vi "SVM_Crossvalidation_FromFile.vi"(8 "error in (no error)":errorcluster) -> (0 "error out":errorcluster, 3 "Predicted labels":dbl[](array[numeric]))   [LabVIEW 2014]
uses:
  Controls/Kernel.ctl
  Libsvm Wrapper/Controls/svm_kernel_type.ctl
  Controls/Options Training.ctl
  Controls/Parameters C_SVC.ctl
  SubVIs/SVM Cross-Validate C_SVC.vi
  <userlib>/_OpenG.lib/error/error.llb/Filter Error Codes (Array)__ogtk.vi
  Libsvm Wrapper/svm_cross_validation.vi
panel:
  in  "Param":T1={"C"=1.0, "weight_label"=[], "weight"=[]}
  in  "Nr Fold":i32=5 caption="Nr fold (LOO)"
  in  "Options":T2={"cache_size"=500.0, "eps"=0.001, "shrinking"=TRUE, "probability"=FALSE}
  in  "Kernel":T3
  out "Logging output":string
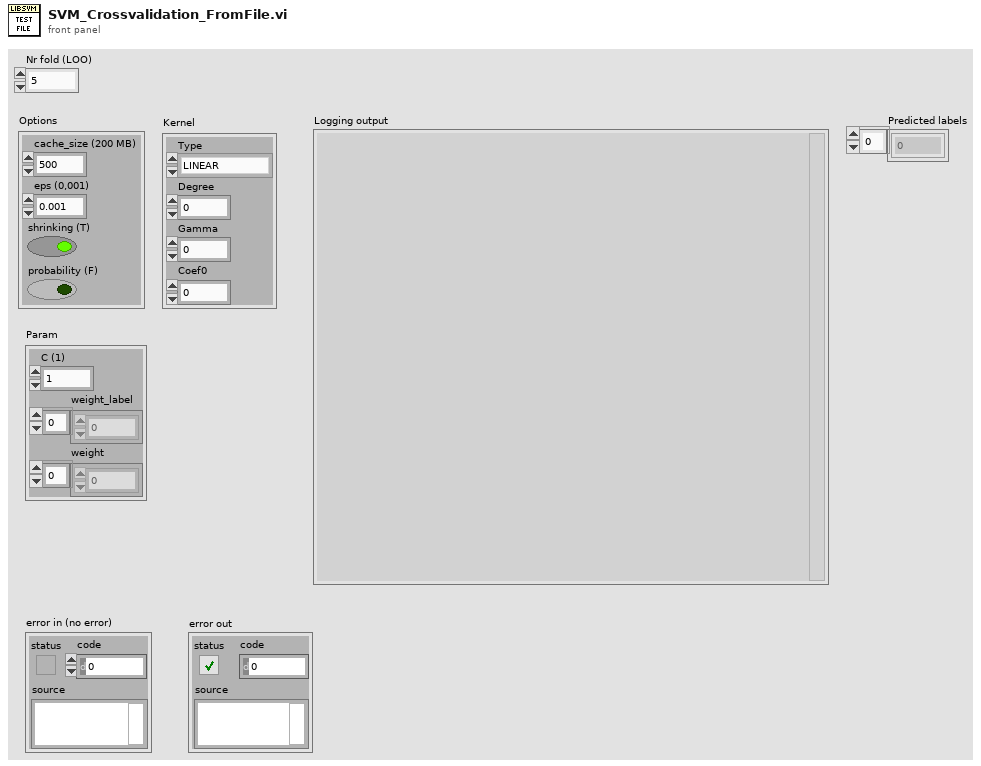
[diagram p1: front panel]
types:
  T1 = typedef "Parameters C_SVC.ctl" = cluster{"C":dbl, "weight_label":i32[], "weight":dbl[]}
  T2 = typedef "Options Training.ctl" = cluster{"cache_size":dbl, "eps":dbl, "shrinking":bool, "probability":bool}
  T3 = typedef "Kernel.ctl" = cluster{"Type":T4, "Degree":i32, "Gamma":dbl, "Coef0":dbl}
  T4 = typedef "svm_kernel_type.ctl" = enum32{"LINEAR", "POLY", "RBF", "SIGMOID", "PRECOMPUTED"}
  T5 = typedef "Logging_MessageQueue.ctl" = cluster{"Time":timestamp, "message":string}
  T6 = typedef "svm_problem.ctl" = cluster{"y":dbl[], "x":cluster{T7[]}[]}
  T7 = typedef "svm_node.ctl" = cluster{"index":i32, "value":dbl}
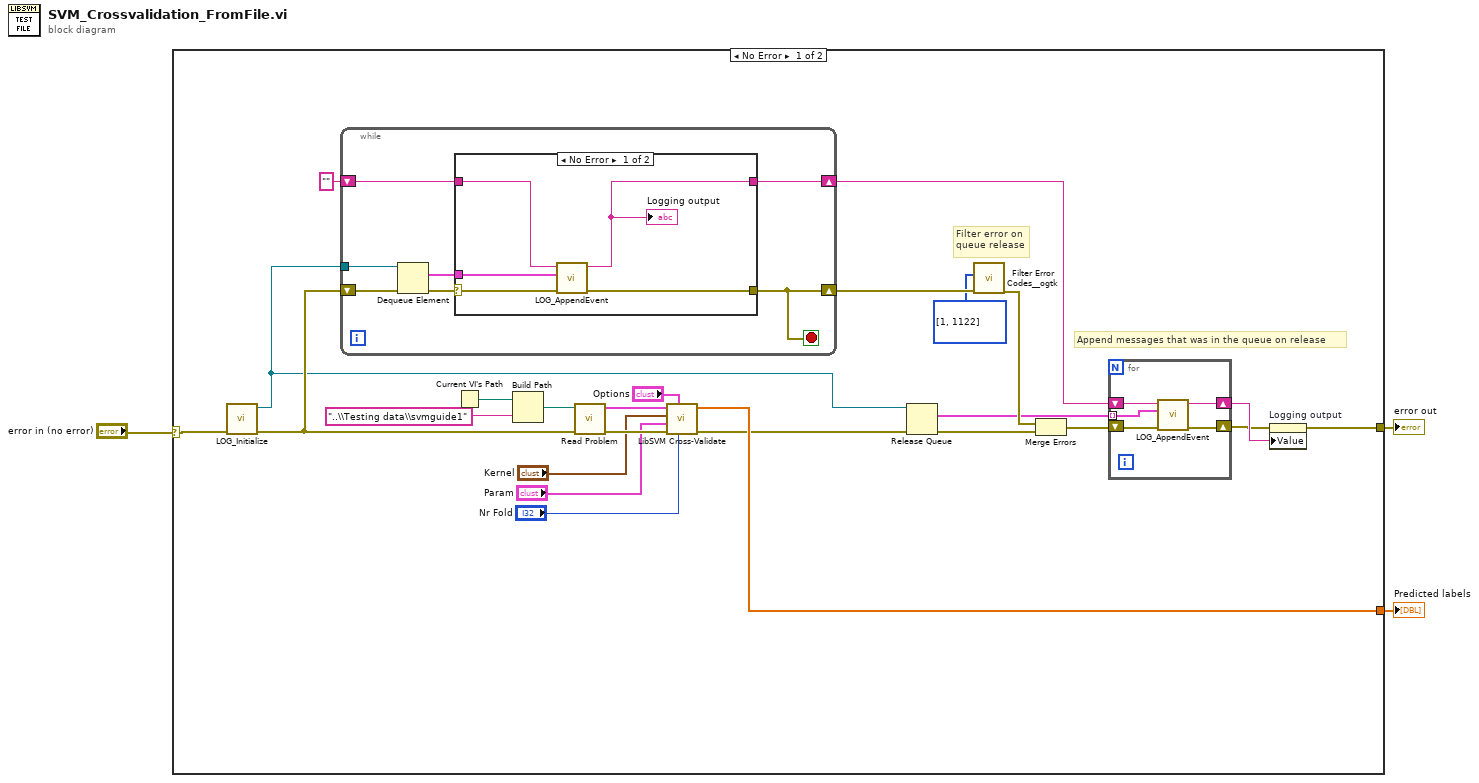
[diagram p0: block diagram]
diagram:
  n1 = case shown="No Error" "error in (no error)" {
    selector: "error in (no error)" -> [w26 w48]
    tunnel: [w14 w48] -> w1
    tunnel: [w11 _] -> w2
    frame No Error {
      # "Append messages that was in the queue on release"
      # "Filter error on\nqueue release"
      n2 = call "LOG_Initialize.vi"("error in (no error)"=w26) -> ("error out"=w24:errorcluster, "Message queue out"=w6:refnum<queue>)  [unwired: 9 in]
      n3 = while {
        tunnel: w6 -> [w40]
        shift-right: [w37] -> w17
        shift-left: "" -> [w36]
        shift-right: [w34] -> w22
        shift-left: w24 -> [w38]
        stop <- w34 stop-if-true
        n4 = Dequeue Element(queue=w40, error in (no error)=w38) -> (element=w39:T5, error out=w35:errorcluster)  [unwired: 1 in, 2 out]
        n5 = case shown="No Error" w35 {
          selector: w35 -> [w42 w47]
          tunnel: w39 -> [w45 _]
          tunnel: [w44 w46] -> w37
          tunnel: w36 -> [w43 w46]
          tunnel: [w41 w47] -> w34
          frame No Error {
            n6 = call "LOG_AppendEvent.vi"("error in (no error)"=w42, "Log Event"=w45, "String in"=w43) -> ("error out"=w41:errorcluster, "String out"=w44:string)  [unwired: 7 in]
            "Logging output" <- w44
          }
          frame Error {
          }
        }
      }
      n7 = Current VI's Path() -> (path=w27:path)
      n8 = Build Path(base path=w27, name or relative path="..\\Testing data\\svmguide1") -> (appended path=w28:path)
      n9 = call "Read Problem.vi"("error in (no error)"=w24, "file path (use dialog)"=w28) -> ("error out"=w12:errorcluster, "svm_problem"=w13:T6)  [unwired: 8 in]
      n10 = call-poly "LibSVM Cross-Validate.vi"("Nr fold"="Nr Fold", "Options"="Options", "error in (no error)"=w12, "Param C_SVC"="Param", "Kernel"="Kernel", "Problem"=w13) -> ("error out"=w7:errorcluster, "Target"=w11:dbl[])  [unwired: 4 in]
      n11 = Release Queue(queue=w6, error in (no error)=w7) -> (remaining elements=w19:T5[], error out=w23:errorcluster)  [unwired: 1 in, 1 out]
      n12 = call-poly <userlib>:"Filter Error Codes__ogtk.vi"("Error In"=w22, "Error Codes to Filter"=i32[] [1, 1122]) -> ("Error Out"=w21:errorcluster)  [unwired: 7 in, 2 out]
      n13 = Merge Errors(w21, w23) -> (w18:errorcluster)
      n14 = for {
        tunnel: w19 -> [w32] mode=indexing
        shift-right: [w30] -> w15
        shift-left: w18 -> [w33]
        shift-right: [w29] -> w16
        shift-left: w17 -> [w31]
        n15 = call "LOG_AppendEvent.vi"("error in (no error)"=w33, "Log Event"=w32, "String in"=w31) -> ("error out"=w30:errorcluster, "String out"=w29:string)  [unwired: 7 in]
      }
      n16 = property on="Logging output" class="Str"(error in=w15, "Value"=w16) -> (error out=w14:errorcluster)  [unwired: 1 in, 1 out]
    }
    frame Error {
    }
  }
  "Predicted labels" <- w2
  "error out" <- w1
